vi "Store Static VI References for Subpanel.vi"(8 "error in (no error)":errorcluster, 11 "Client Config in":refnum<class "Slave Config.lvclass">) -> (0 "error out":errorcluster, 3 "Client Config out":refnum<class "Slave Config.lvclass">)   [LabVIEW 2016, in "Slave Config.lvclass"]
uses:
  <userlib>/Common Components/Slave Configuration/Slave Config.lvclass
  C:/Program Files (x86)/National Instruments/LabVIEW 2016/user.lib/Configuration Dialog Actor/Configuration.lvclass
  <userlib>/Configuration Dialog Actor/Configuration.lvclass
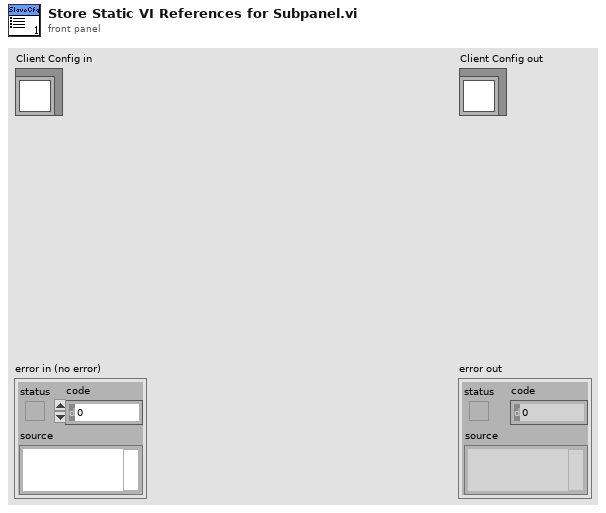
[diagram p1: front panel]
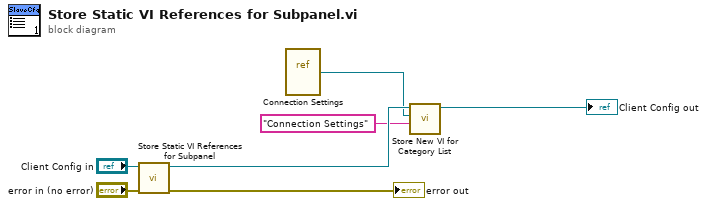
[diagram p0: block diagram]
diagram:
  n1 = call-parent "Store Static VI References for Subpanel.vi"("error in (no error)"="error in (no error)", "Configuration in"="Client Config in") -> ("error out"=→"error out":errorcluster, "Configuration out"=w4:refnum<class "Slave Config.lvclass">)  [unwired: 8 in]
  n2 = vi-ref <userlib>:"Connection Settings.vi"() -> (w1:refnum<vi>)
  n3 = call <userlib>:"Store New VI for Category List.vi"("String"="Connection Settings", "VI Refnum"=w1, "Configuration in"=w4) -> ("Configuration out"=→"Client Config out":refnum<class "Slave Config.lvclass">)  [unwired: 7 in, 1 out]
